vi "Read Picture Control Ref.vi"(8 "error in (no error)":errorcluster, 11 "Reference Control in":refnum<class "Reference Control.lvclass">) -> (0 "error out":errorcluster, 2 "Picture Control Ref":refnum<vi>, 3 "Reference Control out":refnum<class "Reference Control.lvclass">)   [LabVIEW 2016, in "Reference Control.lvclass"]
uses:
  Reference Control.lvclass
  Reference Control.lvclass/Reference Control.ctl
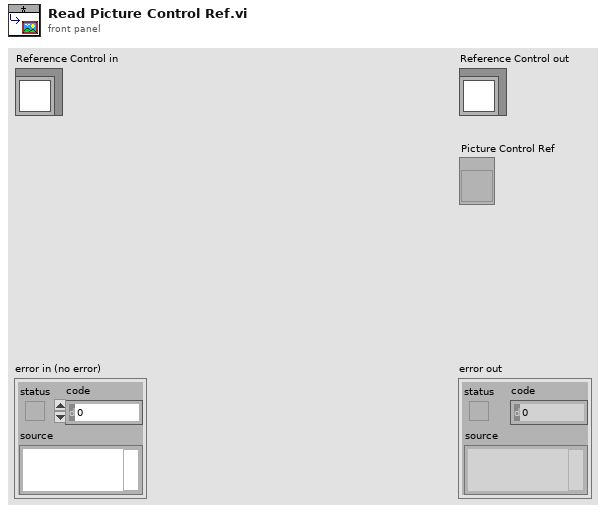
[diagram p1: front panel]
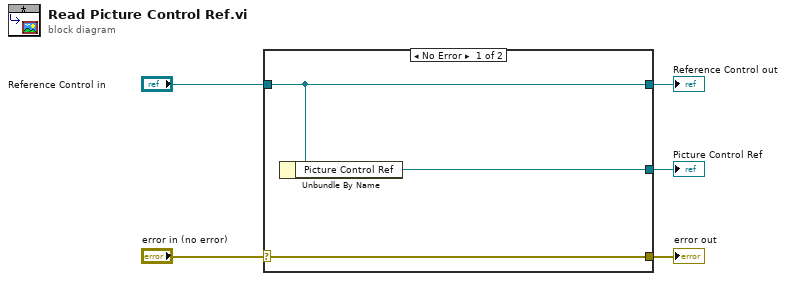
[diagram p0: block diagram]
diagram:
  n1 = case shown="No Error" "error in (no error)" {
    selector: "error in (no error)" -> [w8 w9]
    tunnel: [w8 w9] -> w4
    tunnel: [w7 w10] -> w2
    tunnel: "Reference Control in" -> [w7 w10]
    tunnel: [w6 _] -> w1
    frame No Error {
      n2 = Unbundle By Name(w7) -> ("Picture Control Ref"=w6:refnum<vi>)
    }
    frame Error {
    }
  }
  "error out" <- w4
  "Reference Control out" <- w2
  "Picture Control Ref" <- w1
